vi "readByChannelName.vi"(8 "error in (no error)":errorcluster, 9 "channel_name":string, 10 "Array":refnum<class "rf.lvclass">[](array[class]), 11 "rfArray in":refnum<class "rfArray.lvclass">) -> (0 "error out":errorcluster, 1 "found?":bool, 2 "rf.lvclass":refnum<class "rf.lvclass">, 3 "rfArray out":refnum<class "rfArray.lvclass">)   [LabVIEW 2011, in "Tools.lvlib" / "Scripting.lvlib" / "rfArray.lvclass"]
uses:
  rfArray.lvclass
  Rf Event/rf.lvclass
  DatabaseHelpers/Database Objects/Channel/Channel.lvclass
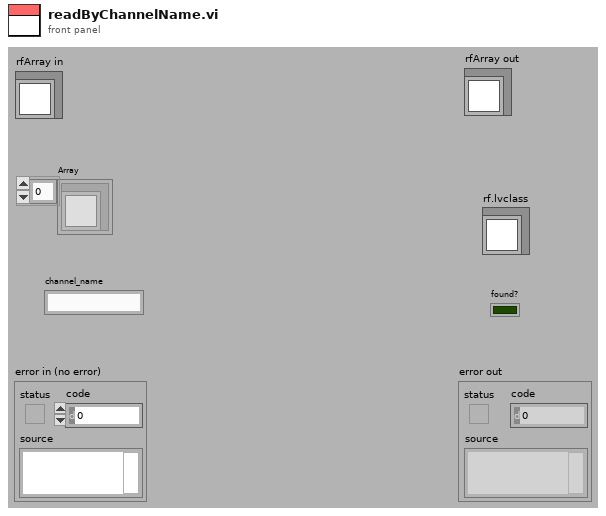
[diagram p1: front panel]
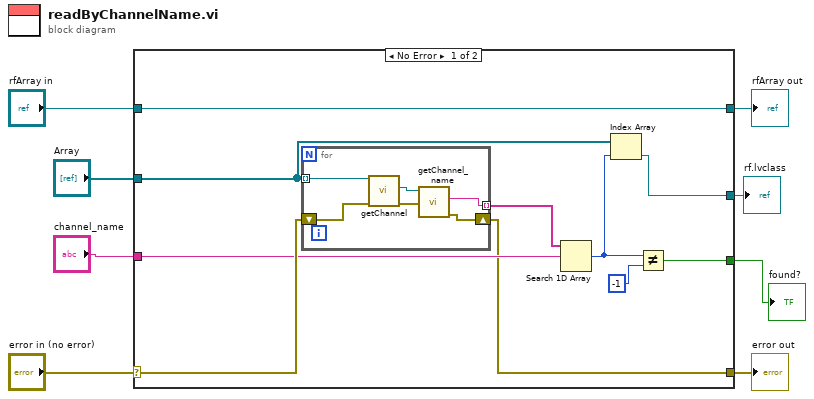
[diagram p0: block diagram]
diagram:
  n1 = case shown="No Error" "error in (no error)" {
    selector: "error in (no error)" -> [w17 w26]
    tunnel: [w12 w26] -> w7
    tunnel: [w18 w25] -> w5
    tunnel: "rfArray in" -> [w18 w25]
    tunnel: "Array" -> [w14 _]
    tunnel: "channel_name" -> [w15 _]
    tunnel: [w13 _] -> w2
    tunnel: [w9 _] -> w1
    frame No Error {
      n2 = for {
        tunnel: w14 -> [w24] mode=indexing
        tunnel: [w22] -> w16 mode=indexing
        shift-right: [w19] -> w12
        shift-left: w17 -> [w20]
        n3 = call-dynamic "getChannel.vi"("error in (no error)"=w20, "ScriptEvent.lvclass in"=w24) -> ("error out"=w21:errorcluster, "Channel.lvclass"=w23:refnum<class "Channel.lvclass">)  [unwired: 7 in, 1 out]
        n4 = call "getChannel_name.vi"("error in (no error)"=w21, "Channel.lvclass in"=w23) -> ("error out"=w19:errorcluster, "channel_name"=w22:string)  [unwired: 7 in, 1 out]
      }
      n5 = Search 1D Array(1D array=w16, element=w15) -> (index of element=w11:i32)  [unwired: 1 in]
      n6 = Index Array(array=w14, index=w11) -> (element=w13:refnum<class "rf.lvclass">)
      n7 = Not Equal?(x=w11, y=-1) -> (x != y?=w9:bool)
    }
    frame Error {
    }
  }
  "error out" <- w7
  "rfArray out" <- w5
  "rf.lvclass" <- w2
  "found?" <- w1
